vi "__para_[CABLE]n.vi"(7 "検索値":string="1", 8 "検索キー列":i32=11, 9 "読み込み配列":string[][](array[string])=[["MixerParam", "4.18", "799", " 2011-02-06  10:16:23", "", "", "", "", "", "", "", "", "", "", "", ""], ["MixerParam", "4.18", "810", " 2011-02-06  10:16:23", "2.02", "50.6", "8.8", "", "", "1", "5", "0", "2.02", "0", "8.96", "0.59"], ["MixerParam", "4.18", "826", " 2011-02-06  10:16:23", "2.04", "50.6", "8.8", "", "", "1", "5", "0", "2.04", "0", "8.96", "0.59"], ["MixerParam", "4.18", "842", " 2011-02-06  10:16:23", "2.06", "50.6", "8.8", "", "", "1", "5", "0", "2.06", "0", "8.96", "0.59"], ["MixerParam", "4.18", "858", " 2011-02-06  10:16:23", "2.08", "50.6", "8.8", "", "", "1", "5", "0", "2.08", "0", "8.96", "0.59"], ["MixerParam", "4.18", "874", " 2011-02-06  10:16:23", "2.1", "50.6", "8.8", "", "", "1", "5", "0", "2.1", "0", "8.96", "0.59"], ["MixerParam", "4.18", "890", " 2011-02-06  10:16:23", "2.12", "50.6", "8.8", "", "", "1", "5", "1", "2.12", "0", "8.96", "0.59"], ["MixerParam", "4.18", "810", " 2011-02-06  10:16:23", "2.02", "50.6", "8.8", "", "", "1", "5", "1", "2.02", "0", "8.96", "0.59"], ["MixerParam", "4.18", "826", " 2011-02-06  10:16:23", "2.04", "50.6", "8.8", "", "", "1", "5", "1", "2.04", "0", "8.96", "0.59"], ["MixerParam", "4.18", "842", " 2011-02-06  10:16:23", "2.06", "50.6", "8.8", "", "", "1", "5", "1", "2.06", "0", "8.96", "0.59"], ["MixerParam", "4.18", "858", " 2011-02-06  10:16:23", "2.08", "50.6", "8.8", "", "", "1", "5", "1", "2.08", "0", "8.96", "0.59"], ["MixerParam", "4.18", "874", " 2011-02-06  10:16:23", "2.1", "50.6", "8.8", "", "", "1", "5", "1", "2.1", "0", "8.96", "0.59"], ["MixerParam", "4.18", "890", " 2011-02-06  10:16:23", "2.12", "50.6", "8.8", "", "", "1", "5", "1", "2.12", "0", "8.96", "0.59"]]) -> (2 "出力配列":string[][](array[string])=[["MixerParam", "4.18", "890", " 2011-02-06  10:16:23", "2.12", "50.6", "8.8", "", "", "1", "5", "1", "2.12", "0", "8.96", "0.59"], ["MixerParam", "4.18", "810", " 2011-02-06  10:16:23", "2.02", "50.6", "8.8", "", "", "1", "5", "1", "2.02", "0", "8.96", "0.59"], ["MixerParam", "4.18", "826", " 2011-02-06  10:16:23", "2.04", "50.6", "8.8", "", "", "1", "5", "1", "2.04", "0", "8.96", "0.59"], ["MixerParam", "4.18", "842", " 2011-02-06  10:16:23", "2.06", "50.6", "8.8", "", "", "1", "5", "1", "2.06", "0", "8.96", "0.59"], ["MixerParam", "4.18", "858", " 2011-02-06  10:16:23", "2.08", "50.6", "8.8", "", "", "1", "5", "1", "2.08", "0", "8.96", "0.59"], ["MixerParam", "4.18", "874", " 2011-02-06  10:16:23", "2.1", "50.6", "8.8", "", "", "1", "5", "1", "2.1", "0", "8.96", "0.59"], ["MixerParam", "4.18", "890", " 2011-02-06  10:16:23", "2.12", "50.6", "8.8", "", "", "1", "5", "1", "2.12", "0", "8.96", "0.59"]])   [LabVIEW 2017]
panel:
  out "検索された列":i32=-1
  out "検索キーの配列":string[](array[string])=["", "0", "0", "0", "0", "0", "1", "1", "1", "1", "1", "1", "1"]
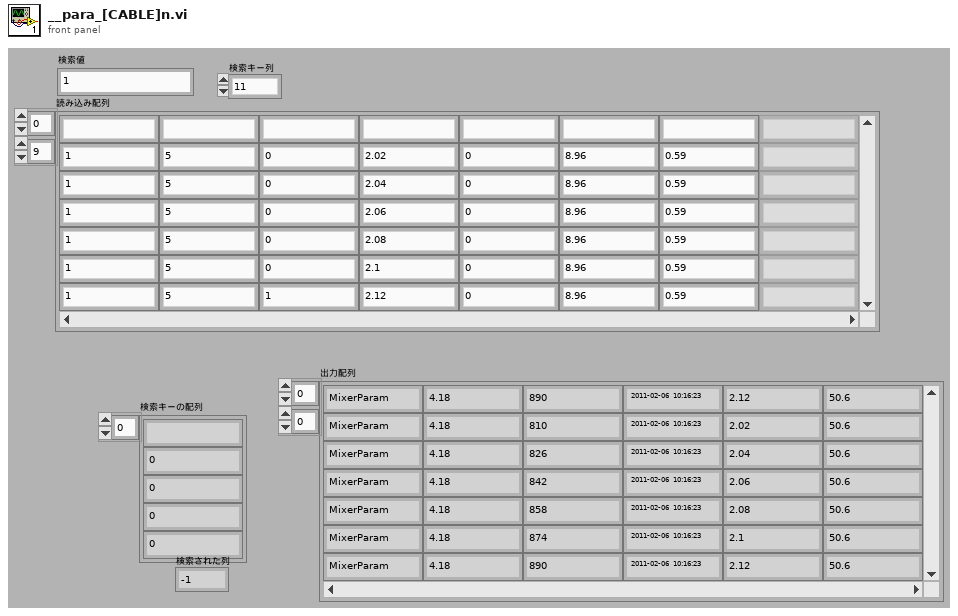
[diagram p1: front panel]
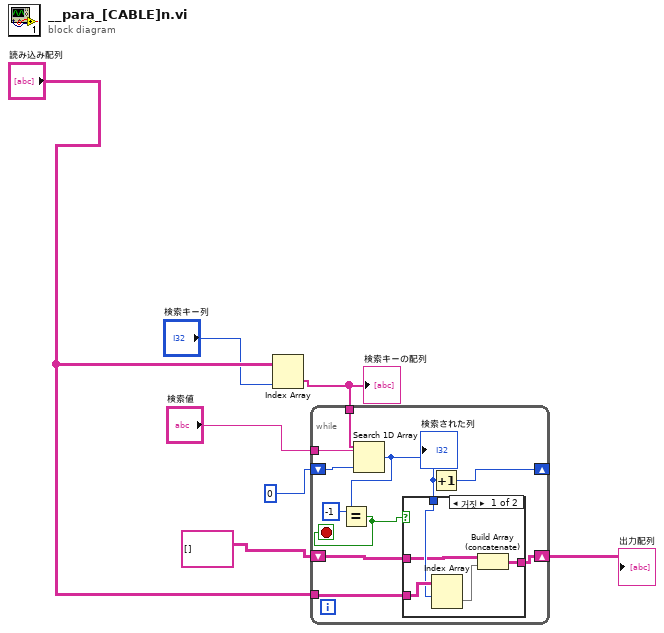
[diagram p0: block diagram]
diagram:
  n1 = Index Array(array="読み込み配列", index (col)="検索キー列") -> (element=w7:string[])  [unwired: 1 in]
  "検索キーの配列" <- w7
  n2 = while {
    tunnel: w7 -> [w17]
    tunnel: "検索値" -> [w16]
    tunnel: "読み込み配列" -> [w15]
    shift-right: [w11] -> _
    shift-left: 0 -> [w13]
    shift-right: [w9] -> w4
    shift-left: string[][] [] -> [w10]
    stop <- w8 stop-if-true
    n3 = Search 1D Array(1D array=w17, element=w16, start index (0)=w13) -> (index of element=w12:i32)
    "検索された列" <- w12
    n4 = Equal?(x=w12, y=-1) -> (x = y?=w8:bool)
    n5 = case shown="거짓" w8 {
      tunnel: w15 -> [w22 _]
      tunnel: w12 -> [w21 _]
      tunnel: w10 -> [w20 w23]
      tunnel: [w18 w23] -> w9
      frame False {
        n6 = Index Array(array=w22, index (row)=w21) -> (element=w19:string[])  [unwired: 1 in]
        n7 = Build Array (concatenate)(w20, w19) -> (w18:string[][])
      }
      frame True {
      }
    }
    n8 = Increment(x=w12) -> (x+1=w11:i32)
  }
  "出力配列" <- w4
